vi "Main_2.vi"() -> ()   [LabVIEW 2016]
uses:
  <vilib>/Platform/TimedLoop/XDataNode/timing_clust.ctl
  <vilib>/Platform/TimedLoop/XDataNode/nitl_modes.ctl
  <vilib>/Platform/TimedLoop/XDataNode/wakeup.ctl
  <vilib>/Instr/_visa.llb/VISA Configure Serial Port (Instr).vi
  <vilib>/httpClient/POSTBuffer.vi
  <vilib>/platform/TimedLoop/XDataNode/XDataNode.xnode
  <vilib>/Platform/TimedLoop/XDataNode/XDNodeRunTimeDep.lvlib
  <vilib>/httpClient/LabVIEWHTTPClient.lvlib
panel:
  in  "?":enum32{"Battery", "Capacitor"}(tab)
  in  "?":enum32{"Rem Capacity", "Full Capacity"}(tab)
  out "BATTERY REM CAPACITY 4":dbl
  out "BATTERY REM CAPACITY 3":dbl
  out "BATTERY REM CAPACITY 2":dbl
  out "BATTERY REM CAPACITY 1":dbl
  out "BATTERY REM CAPACITY 5":dbl
  out "BATTERY FULL CAPACITY 4":dbl
  out "BATTERY FULL CAPACITY 3":dbl
  out "BATTERY FULL CAPACITY 2":dbl
  out "BATTERY FULL CAPACITY 1":dbl
  out "BATTERY FULL CAPACITY 5":dbl
  in  "?":T1(tab)
  out "BATTERY VOLTAGE 3":dbl
  out "BATTERY VOLTAGE 2":dbl
  out "BATTERY VOLTAGE 1":dbl
  out "BATTERY VOLTAGE 4":dbl
  out "Slide 4":u8(slide) scale=0.0..100.0
  out "Slide":u8(slide) scale=0.0..100.0
  out "Slide 2":u8(slide) scale=0.0..100.0
  out "Slide 3":u8(slide) scale=0.0..100.0
  out "BATTERY VOLTAGE 5":dbl
  out "Slide 8":u8(slide) scale=0.0..100.0
  out "Slide 7":u8(slide) scale=0.0..100.0
  out "Slide 6":u8(slide) scale=0.0..100.0
  out "Slide 5":u8(slide) scale=0.0..100.0
  out "BATTERY CURRENT 1":dbl
  out "BATTERY CURRENT 2":dbl
  out "BATTERY CURRENT 3":dbl
  out "BATTERY CURRENT 4":dbl
  out "BATTERY CURRENT 5":dbl
  in  "LO2-REL 2":bool
  in  "LO2-REL 1":bool
  in  "LO1-REL 2":bool
  in  "LO1-REL 1":bool
  in  "SUPERCAP-GATE 6":bool
  in  "BATT-GATE 4":bool
  in  "BATT-GATE 3":bool
  in  "BATT-GATE 5":bool
  in  "BATT-GATE 1":bool
  in  "BATT-GATE 2":bool
  out "Power Switch Led":bool
  out "Power Button State":dbl
  in  "Batter data send url":string
  in  "control battery url":string
  in  "VISA resource name":refnum<visa-resource-name>
  in  "Continuous Measurement":bool
  in  "?":enum32{"Temperature", "Power"}(tab)
  out "BATTERY TEMP: 4":dbl
  out "BATTERY TEMP: 3":dbl
  out "BATTERY TEMP: 2":dbl
  out "BATTERY TEMP: 1":dbl
  out "BATTERY TEMP: 5":dbl
  out "BATTERY POWER 5":dbl
  out "BATTERY POWER 4":dbl
  out "BATTERY  POWER 3":dbl
  out "BATTERY POWER 2":dbl
  out "BATTERY POWER 1":dbl
  in  "?":T2(tab)
  out "BATTERY RATED ENERGY 1":dbl
  out "BATTERY RATED ENERGY 2":dbl
  out "BATTERY RATED ENERGY 3":dbl
  out "BATTERY RATED ENERGY 4":dbl
  out "BATTERY RATED ENERGY 5":dbl
  out "BATTERY MAX ENERGY 4":dbl
  out "BATTERY MAX ENERGY 3":dbl
  out "BATTERY MAX ENERGY 2":dbl
  out "BATTERY MAX ENERGY 1":dbl
  out "BATTERY MAX ENERGY 5":dbl
  out "BATTERY AVAIL ENERGY 4":dbl
  out "BATTERY AVAIL ENERGY 3":dbl
  out "BATTERY AVAIL ENERGY 2":dbl
  out "BATTERY AVAIL ENERGY 1":dbl
  out "BATTERY AVAIL ENERGY 5":dbl
  in  "?":enum32{"Voltage", "Temperature", "TAP Voltage"}(tab)
  out "Vertical Progress Bar 6":u8(slide) scale=0.0..100.0
  out "Vertical Progress Bar 5":u8(slide) scale=0.0..100.0
  out "Vertical Progress Bar 4":u8(slide) scale=0.0..100.0
  out "Vertical Progress Bar 3":u8(slide) scale=0.0..100.0
  out "Vertical Progress Bar 2":u8(slide) scale=0.0..100.0
  out "Vertical Progress Bar":u8(slide) scale=0.0..100.0
  out "?":u8(slide) scale=0.0..100.0
  out "VOLT-CAP-6":dbl
  out "VOLT-CAP-5":dbl
  out "VOLT-CAP-4":dbl
  out "VOLT-CAP-3":dbl
  out "VOLT-CAP-2":dbl
  out "VOLT-CAP-1":dbl
  out "Temp_1":dbl(slide) scale=0.0..100.0
  out "Temp_2":dbl(slide) scale=0.0..100.0
  out "Temp_3":dbl(slide) scale=0.0..100.0
  out "Temp_4":dbl(slide) scale=0.0..100.0
  out "Temp_5":dbl(slide) scale=0.0..100.0
  out "Temp_6":dbl(slide) scale=0.0..100.0
  out "MOD 6":bool
  out "MOD 5":bool
  out "TAP 7":dbl(slide) scale=0.0..100.0
  out "TAP 8":dbl(slide) scale=0.0..100.0
  out "TAP 9":dbl(slide) scale=0.0..100.0
  out "TAP 10":dbl(slide) scale=0.0..100.0
  out "TAP 11":dbl(slide) scale=0.0..100.0
  out "TAP 12":dbl(slide) scale=0.0..100.0
  out "TAP 13":dbl(slide) scale=0.0..100.0
  out "TAP 14":dbl(slide) scale=0.0..100.0
  out "TAP 15":dbl(slide) scale=0.0..100.0
  out "TAP 16":dbl(slide) scale=0.0..100.0
  out "TAP 17":dbl(slide) scale=0.0..100.0
  out "TAP 18":dbl(slide) scale=0.0..100.0
  out "MOD 4":bool
  out "TAP 19":dbl(slide) scale=0.0..100.0
  out "TAP 20":dbl(slide) scale=0.0..100.0
  out "TAP 4_":dbl(slide) scale=0.0..100.0
  out "TAP 4_3":dbl(slide) scale=0.0..100.0
  out "TAP 4_2":dbl(slide) scale=0.0..100.0
  out "TAP 4_1":dbl(slide) scale=0.0..100.0
  out "MOD 3":bool
  out "MOD 2":bool
  out "MOD 1":bool
  out "TAP 3_3":dbl(slide) scale=0.0..12.0
  out "TAP 3_1":dbl(slide) scale=0.0..5.0
  out "TAP 3_2":dbl(slide) scale=0.0..8.0
  out "TAP 3_6":dbl(slide) scale=0.0..25.0
  out "TAP 3_4":dbl(slide) scale=0.0..16.0
  out "TAP 3_5":dbl(slide) scale=0.0..20.0
  out "TAP 2_6":dbl(slide) scale=0.0..25.0
  out "TAP 2_5":dbl(slide) scale=0.0..20.0
  out "TAP 2_4":dbl(slide) scale=0.0..16.0
  out "TAP 2_3":dbl(slide) scale=0.0..12.0
  out "TAP 2_2":dbl(slide) scale=0.0..8.0
  out "TAP 2_1":dbl(slide) scale=0.0..5.0
  out "TAP 1_5":dbl(slide) scale=0.0..20.0
  out "TAP 1_4":dbl(slide) scale=0.0..16.0
  out "TAP 1_6":dbl(slide) scale=0.0..25.0
  out "TAP 1_3":dbl(slide) scale=0.0..12.0
  out "TAP 1_2":dbl(slide) scale=0.0..8.0
  out "TAP 1_1":dbl(slide) scale=0.0..5.0
  in  "?":bool
  in  "Stop RT":bool
  out "TAP Voltages":cluster{dbl[], dbl[]}[](graph)
  out "Counter Register":dbl
  out "Total Received":u32
  out "Module's Voltages":cluster{dbl[], dbl[]}[](graph)
  in  "Transmit Frame":T3={"timestamp high"=0, "timestamp low"=0, "identifier"=18, "type"=enum."Data Frame", "info A"=0, "info B"=0, "data length"=8, "data"=[0, 0, 0, 0, 0, 0, 0, 0]} {"identifier" format="%x"; "data" format="%.0x"}
  # "https://aertcsmartgrid.onrender.com/receive-data"
  # "https://aertcsmartgrid.onrender.com/get-btcontrol"
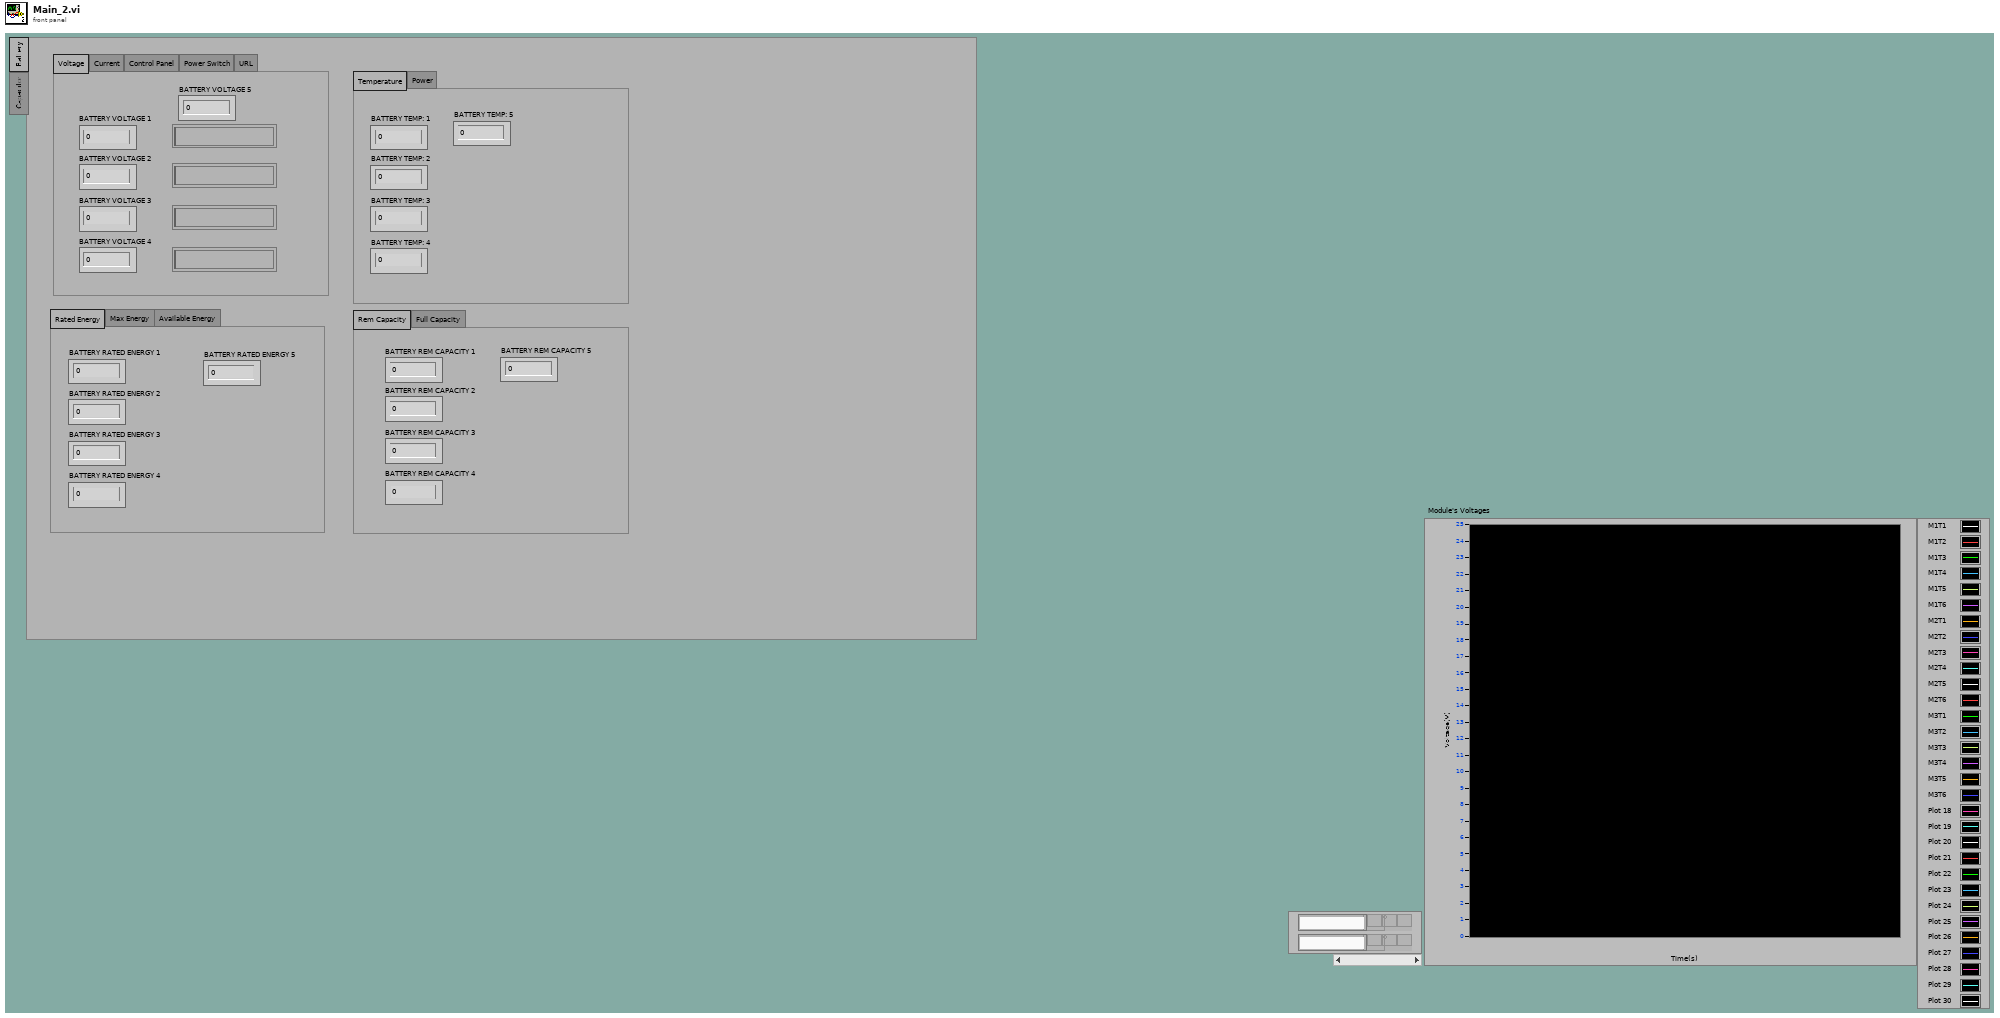
[diagram p1: front panel]
types:
  T1 = enum32{"Voltage", "Current", "Control Panel", "Power Switch", "URL"}
  T2 = enum32{"Rated Energy", "Max Energy", "Available Energy"}
  T3 = cluster{"timestamp high":u32, "timestamp low":u32, "identifier":u32, "type":enum8{"Data Frame", "Remote Frame", "(reserved)", "(reserved) ", "(reserved)  ", "(reserved)   ", "Bus Error", "Transceiver Fault"}, "info A":u8, "info B":u8, "data length":u8, "data":u8[]}
  T4 = typedef "XDNodeRunTimeDep.lvlib/timing_clust.ctl" = cluster{"Expected End [f-1]":u64, "Actual End [f-1]":u64, "Finished Late? [f-1]":bool, "Expected End [i-1]":u64, "Actual End [i-1]":u64, "Finished Late? [i-1]":bool, "Expected Start [i]":u64, "Actual Start [i]":u64, "Expected Start [f]":u64, "Actual Start [f]":u64, "Source Name":string, "Structure Name":string, "Period":i64, "Deadline":i64, "Offset":i64, "Start":i64, "Priority":i32, "Timeout":i32, "Mode":T5, "Wakeup Reason":T6, "Error":errorcluster, "Source Type":string, "Secondary Source Type":string, "Global End Time":u64, "Global Start Time":u64, "Frame Duration":u64, "Iteration Duration":u64, "Assigned CPU":i32, "I/O Scan Engine Mode":u32}
  T5 = typedef "XDNodeRunTimeDep.lvlib/nitl_modes.ctl" = enum32{"No Change", "Process missed periods, maintain original phase", "Discard missed periods, maintain original phase", "Process missed periods, ignore original phase", "Discard missed periods, ignore original phase"}
  T6 = typedef "XDNodeRunTimeDep.lvlib/wakeup.ctl" = enum32{"Normal", "Aborted", "Asynchronous wakeup", "Timing source error", "Timed loop error", "Timeout"}
  T7 = typedef "LabVIEWHTTPClient.lvlib/ClientHandle.ctl" = refnum<k1>
  T8 = cluster{"unsigned byte array[0]":u8, "unsigned byte array[1]":u8, "unsigned byte array[2]":u8, "unsigned byte array[3]":u8, "unsigned byte array[4]":u8, "unsigned byte array[5]":u8, "unsigned byte array[6]":u8, "unsigned byte array[7]":u8, "unsigned byte array[8]":u8}
  T9 = cluster{"data[0]":u8, "data[1]":u8, "data[2]":u8, "data[3]":u8, "data[4]":u8, "data[5]":u8, "data[6]":u8, "data[7]":u8, "data[8]":u8}
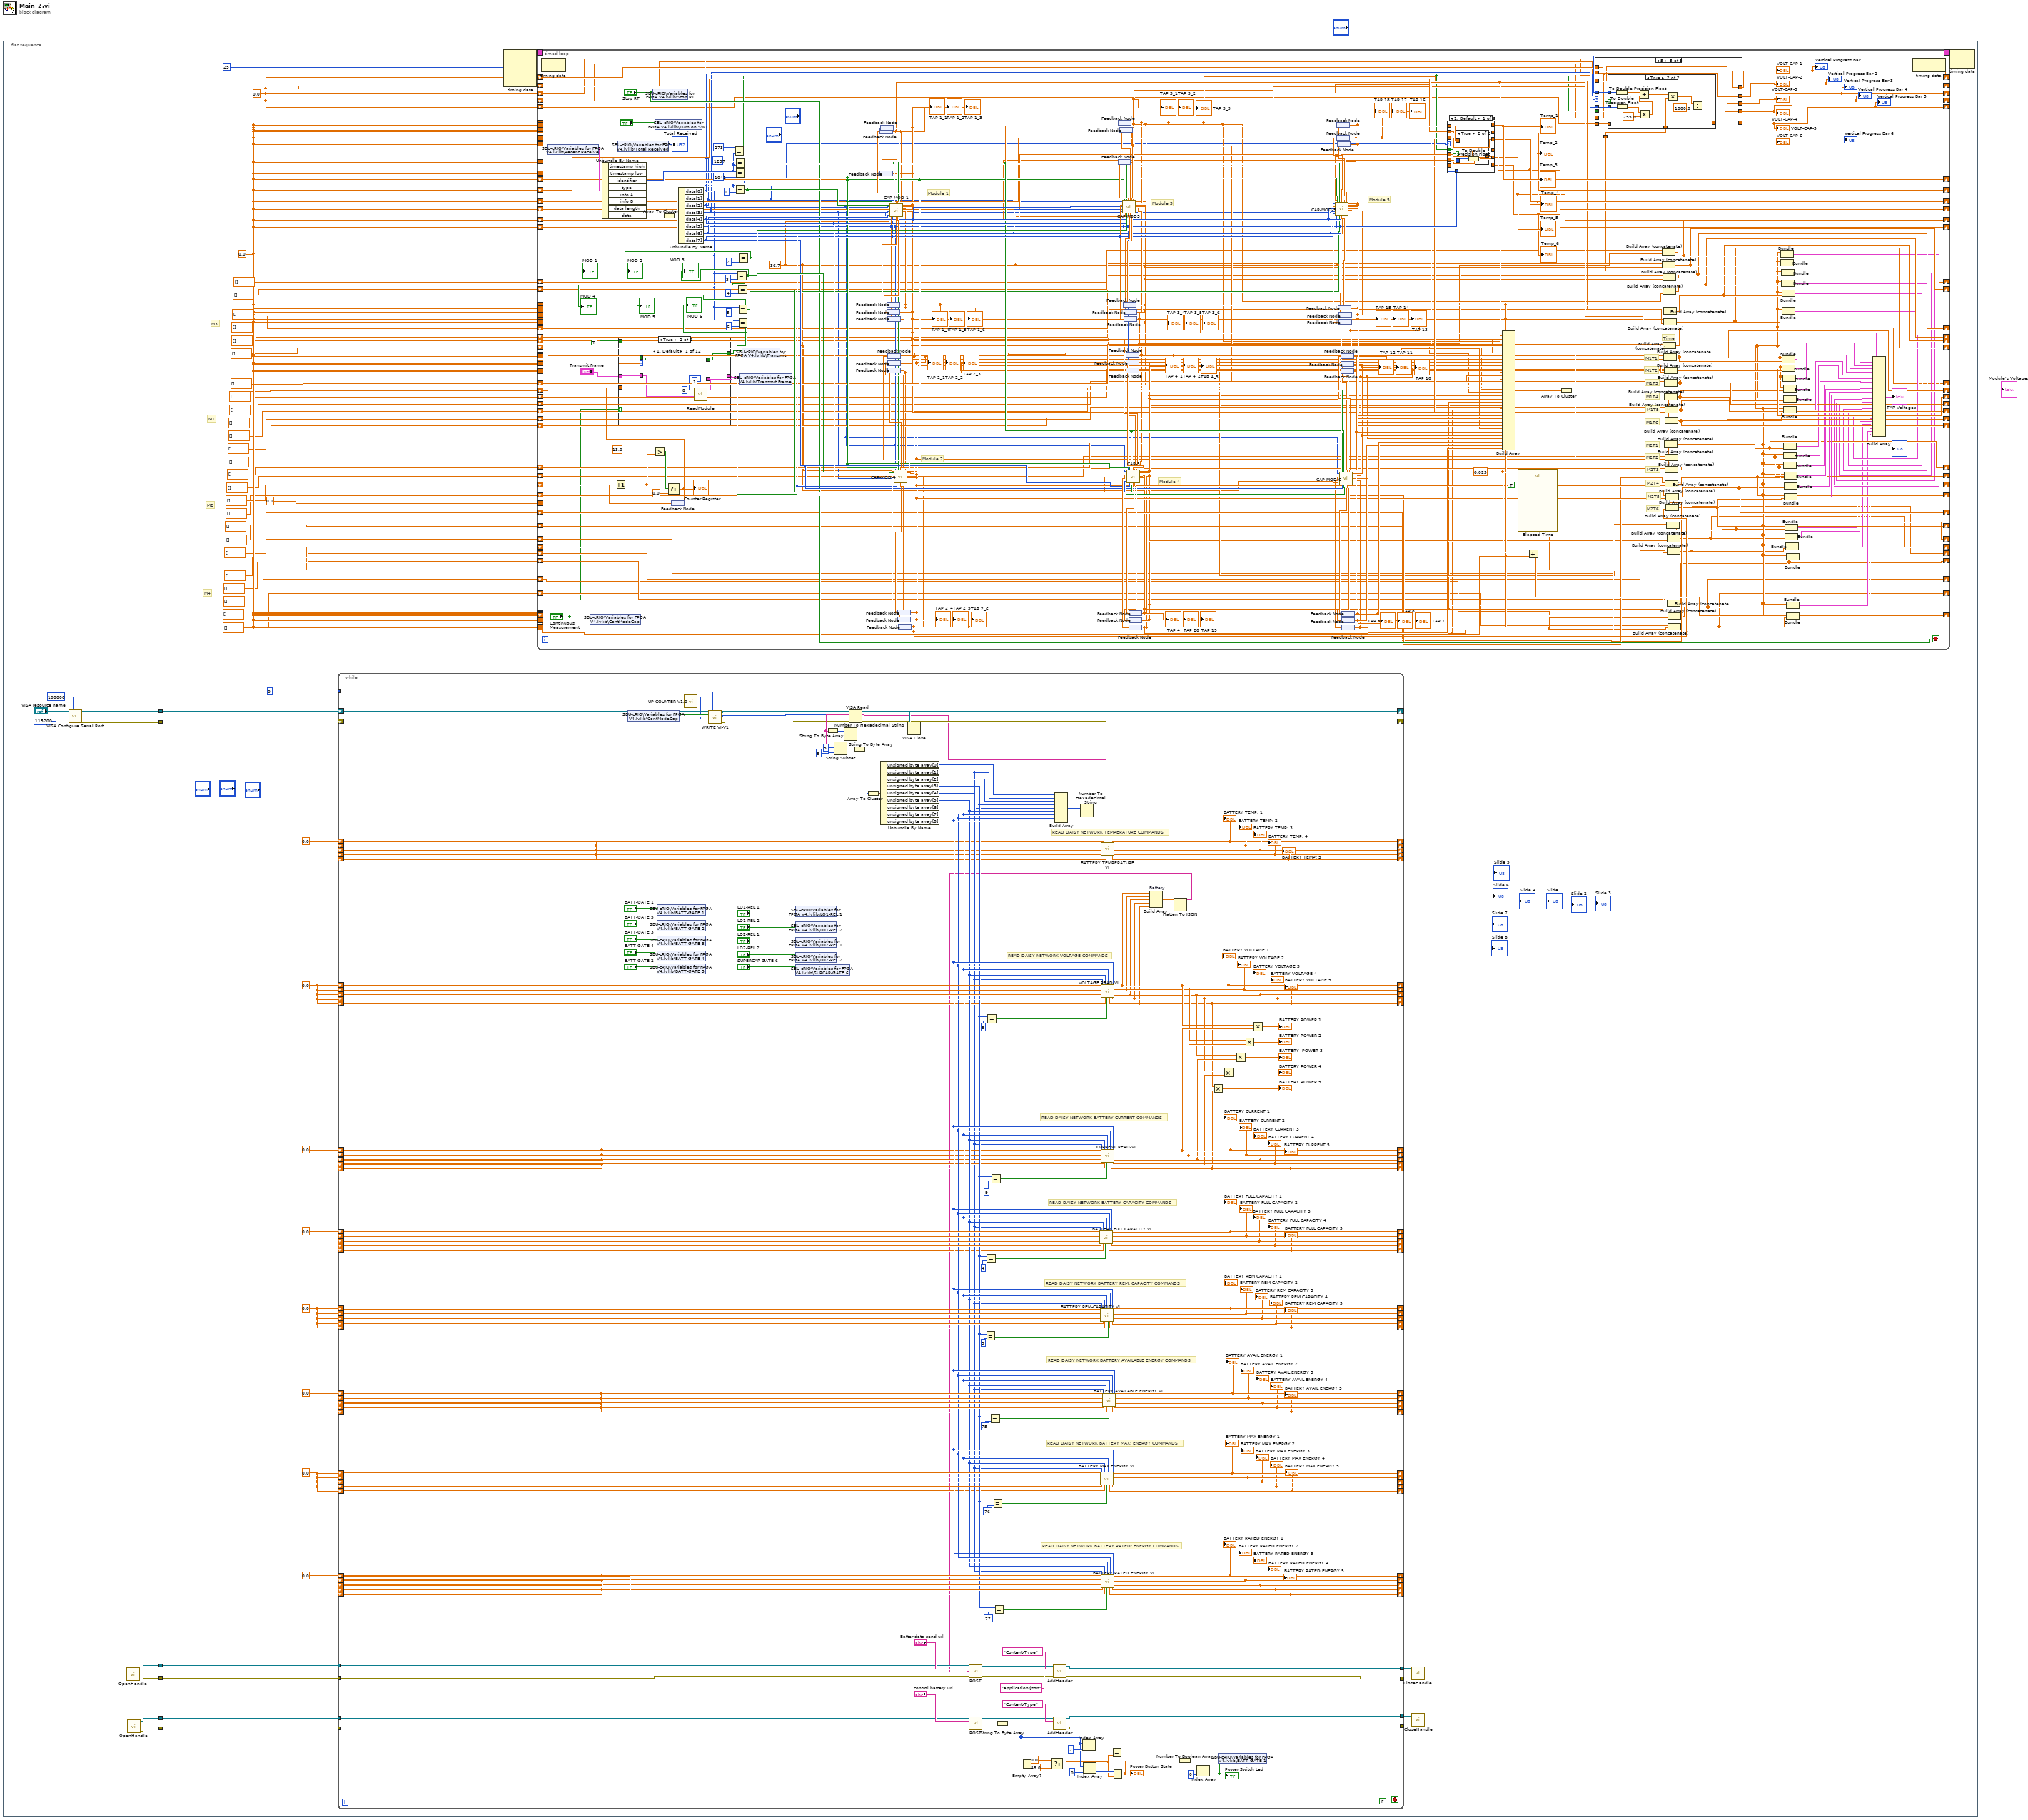
[diagram p0: block diagram]
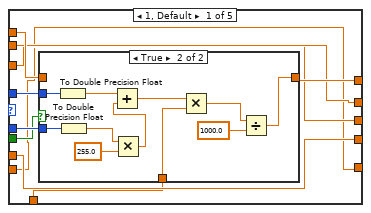
[diagram p2: hidden frame]
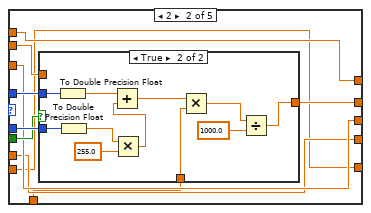
[diagram p4: hidden frame]
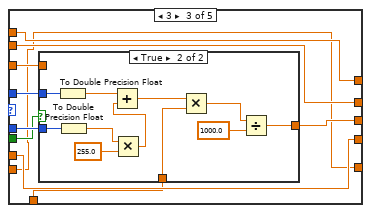
[diagram p6: hidden frame]
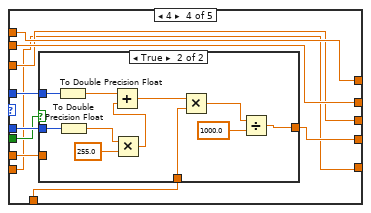
[diagram p8: hidden frame]
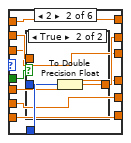
[diagram p12: hidden frame]
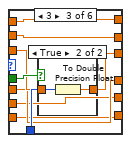
[diagram p14: hidden frame]
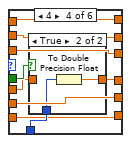
[diagram p16: hidden frame]
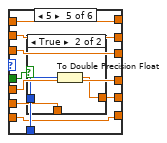
[diagram p18: hidden frame]
diagram:
  n1 = flat-sequence {
    tunnel: [w12] -> w6
    tunnel: [w11] -> w5
    tunnel: [w10] -> w4
    tunnel: [w9] -> w3
    tunnel: [w8] -> w2
    tunnel: [w7] -> w1
    tunnel: w6 -> [w34]
    tunnel: w5 -> [w33]
    tunnel: w4 -> [w19]
    tunnel: w3 -> [w18]
    tunnel: w2 -> [w17]
    tunnel: w1 -> [w16]
    frame #0 {
      n2 = call-poly "VISA Configure Serial Port"("VISA resource name"="VISA resource name", "timeout (10sec)"=u32 100000, "baud rate (9600)"=u32 115200) -> ("VISA resource name out"=w12:refnum<visa-resource-name>, "error out"=w11:errorcluster)  [unwired: 11 in]
      n3 = call <vilib>:"OpenHandle.vi"() -> ("client handle out"=w10:T7, "error out"=w9:errorcluster)  [unwired: 14 in]
      n4 = call <vilib>:"OpenHandle.vi"() -> ("client handle out"=w8:T7, "error out"=w7:errorcluster)  [unwired: 14 in]
    }
    frame #1 {
      w30 = 0.0
      w24 = 0.0
      w32 = 0.0
      w27 = 0.0
      w26 = 0.0
      w28 = 0.0
      w25 = 0.0
      w29 = 0.0
      w31 = 0.0
      w62 = 0.0
      # "M4"
      # "M3"
      # "M2"
      # "M1"
      n5 = while {
        shift-right: [w117] -> w37
        shift-left: w34 -> [w75]
        shift-right: [w116] -> w36
        shift-left: w33 -> [w69]
        tunnel: 0 -> [w73]
        shift-right: [w82] -> _
        shift-left: w31 -> [w173]
        shift-right: [w81] -> _
        shift-left: w31 -> [w174]
        shift-right: [w80] -> _
        shift-left: w31 -> [w175]
        shift-right: [w79] -> _
        shift-left: w31 -> [w176]
        shift-right: [w215] -> _
        shift-left: w29 -> [w216]
        shift-right: [w214] -> _
        shift-left: w29 -> [w172]
        shift-right: [w213] -> _
        shift-left: w29 -> [w211]
        shift-right: [w212] -> _
        shift-left: w29 -> [w210]
        shift-right: [w205] -> _
        shift-left: w25 -> [w209]
        shift-right: [w204] -> _
        shift-left: w25 -> [w208]
        shift-right: [w203] -> _
        shift-left: w25 -> [w207]
        shift-right: [w202] -> _
        shift-left: w25 -> [w206]
        shift-right: [w201] -> _
        shift-left: w28 -> [w197]
        shift-right: [w200] -> _
        shift-left: w28 -> [w196]
        shift-right: [w199] -> _
        shift-left: w28 -> [w195]
        shift-right: [w198] -> _
        shift-left: w28 -> [w194]
        shift-right: [w189] -> _
        shift-left: w26 -> [w193]
        shift-right: [w188] -> _
        shift-left: w26 -> [w192]
        shift-right: [w187] -> _
        shift-left: w26 -> [w191]
        shift-right: [w186] -> _
        shift-left: w26 -> [w190]
        shift-right: [w181] -> _
        shift-left: w27 -> [w185]
        shift-right: [w180] -> _
        shift-left: w27 -> [w184]
        shift-right: [w179] -> _
        shift-left: w27 -> [w183]
        shift-right: [w178] -> _
        shift-left: w27 -> [w182]
        shift-right: [w160] -> _
        shift-left: w30 -> [w163]
        shift-right: [w158] -> _
        shift-left: w30 -> [w162]
        shift-right: [w157] -> _
        shift-left: w30 -> [w161]
        shift-right: [w156] -> _
        shift-left: w30 -> [w164]
        shift-right: [w78] -> _
        shift-left: w31 -> [w152]
        shift-right: [w148] -> _
        shift-left: w30 -> [w150]
        shift-right: [w146] -> _
        shift-left: w29 -> [w147]
        shift-right: [w144] -> _
        shift-left: w25 -> [w145]
        shift-right: [w142] -> _
        shift-left: w28 -> [w143]
        shift-right: [w140] -> _
        shift-left: w26 -> [w141]
        shift-right: [w138] -> _
        shift-left: w27 -> [w139]
        shift-right: [w132] -> _
        shift-left: w24 -> [w137]
        shift-right: [w131] -> _
        shift-left: w24 -> [w136]
        shift-right: [w130] -> _
        shift-left: w24 -> [w135]
        shift-right: [w129] -> _
        shift-left: w24 -> [w134]
        shift-right: [w114] -> _
        shift-left: w24 -> [w133]
        tunnel: [w91] -> w23
        tunnel: [w90] -> w22
        tunnel: [w89] -> w21
        tunnel: [w88] -> w20
        tunnel: w19 -> [w87]
        tunnel: w18 -> [w86]
        tunnel: w17 -> [w85]
        tunnel: w16 -> [w84]
        stop <- FALSE stop-if-true
        # "READ DAISY NETWORK TEMPERATURE COMMANDS"
        # "READ DAISY NETWORK BATTERY CURRENT COMMANDS"
        # "READ DAISY NETWORK BATTERY RATED: ENERGY COMMANDS"
        # "READ DAISY NETWORK BATTERY MAX: ENERGY COMMANDS"
        # "READ DAISY NETWORK BATTERY AVAILABLE ENERGY COMMANDS"
        # "READ DAISY NETWORK BATTERY REM: CAPACITY COMMANDS"
        # "READ DAISY NETWORK BATTERY CAPACITY COMMANDS"
        # "READ DAISY NETWORK VOLTAGE COMMANDS"
        n6 = shared-variable "SBU-cRIO\\Variables for FPGA V4.lvlib\\ContModeCap"() -> (w72:bool)  [unwired: 1 in, 1 out]
        n7 = shared-variable "SBU-cRIO\\Variables for FPGA V4.lvlib\\BATT-GATE 1"("BATT-GATE 1") -> ()  [unwired: 1 in, 1 out]
        n8 = shared-variable "SBU-cRIO\\Variables for FPGA V4.lvlib\\BATT-GATE 2"("BATT-GATE 5") -> ()  [unwired: 1 in, 1 out]
        n9 = shared-variable "SBU-cRIO\\Variables for FPGA V4.lvlib\\BATT-GATE 3"("BATT-GATE 3") -> ()  [unwired: 1 in, 1 out]
        n10 = shared-variable "SBU-cRIO\\Variables for FPGA V4.lvlib\\BATT-GATE 4"("BATT-GATE 4") -> ()  [unwired: 1 in, 1 out]
        n11 = shared-variable "SBU-cRIO\\Variables for FPGA V4.lvlib\\BATT-GATE 5"("BATT-GATE 2") -> ()  [unwired: 1 in, 1 out]
        n12 = call "UP-COUNTER-V1.0.vi"() -> ("COUNT"=w68:u32)  [unwired: 11 in]
        n13 = call "WRITE VI-V1.vi"("Numeric"=w73, "error in (no error)"=w69, "COUNT"=w68, "BATTERY MEASUREMENTS"=w72, "VISA Refnum in"=w75) -> ("error out"=w70:errorcluster, "Bytes at Port"=w71:u32, "VISA Refnum out"=w74:refnum<visa-resource-name>)  [unwired: 4 in]
        n14 = shared-variable "SBU-cRIO\\Variables for FPGA V4.lvlib\\LO1-REL 1"("LO1-REL 1") -> ()  [unwired: 1 in, 1 out]
        n15 = shared-variable "SBU-cRIO\\Variables for FPGA V4.lvlib\\LO1-REL 2"("LO1-REL 2") -> ()  [unwired: 1 in, 1 out]
        n16 = shared-variable "SBU-cRIO\\Variables for FPGA V4.lvlib\\LO2-REL 1"("LO2-REL 1") -> ()  [unwired: 1 in, 1 out]
        n17 = shared-variable "SBU-cRIO\\Variables for FPGA V4.lvlib\\LO2-REL 2"("LO2-REL 2") -> ()  [unwired: 1 in, 1 out]
        n18 = shared-variable "SBU-cRIO\\Variables for FPGA V4.lvlib\\SUPCAP-GATE 6"("SUPERCAP-GATE 6") -> ()  [unwired: 1 in, 1 out]
        n19 = VISA Read(VISA resource name=w74, byte count=w71, error in (no error)=w70) -> (VISA resource name out=w117:refnum<visa-resource-name>, read buffer=w115:string, error out=w116:errorcluster)  [unwired: 1 out]
        n20 = String To Byte Array(string=w115) -> (unsigned byte array=w217:u8[])
        n21 = String Subset(string=w115, offset (0)=5, length (rest)=8 ("length (rest)")) -> (substring=w234:string)
        n22 = Number To Hexadecimal String(2:w217) -> ()  [unwired: 1 in, 1 out]
        n23 = String To Byte Array(string=w234) -> (unsigned byte array=w233:u8[])
        n24 = Array To Cluster(array=w233) -> (cluster=w229:T8)
        n25 = Unbundle By Name(w229) -> ("unsigned byte array[0]"=w232:u8, "unsigned byte array[1]"=w151:u8, "unsigned byte array[2]"=w231:u8, "unsigned byte array[3]"=w165:u8, "unsigned byte array[4]"=w118:u8, "unsigned byte array[5]"=w166:u8, "unsigned byte array[6]"=w167:u8, "unsigned byte array[7]"=w168:u8, "unsigned byte array[8]"=w169:u8)
        n26 = call-poly <vilib>:"POST.vi"("client handle"=w85, "url"="control battery url", "error in (no error)"=w84) -> ("client handle out"=w106:T7, "body"=w102:string, "error out"=w105:errorcluster)  [unwired: 9 in, 1 out]
        n27 = Equal?(x=w165, y=u32 3) -> (x = y?=w224:bool)
        n28 = Equal?(x=w165, y=u32 4) -> (x = y?=w226:bool)
        n29 = Equal?(x=w165, y=u32 8) -> (x = y?=w177:bool)
        n30 = Equal?(x=w165, y=u32 75) -> (x = y?=w222:bool)
        n31 = Equal?(x=w165, y=u32 9) -> (x = y?=w170:bool)
        n32 = Equal?(x=w165, y=u32 76) -> (x = y?=w220:bool)
        n33 = Equal?(x=w165, y=u32 77) -> (x = y?=w218:bool)
        n34 = String To Byte Array(string=w102) -> (unsigned byte array=w98:u8[])
        n35 = Empty Array?(array=w98) -> (empty?=w99:bool)
        n36 = Select(t=0.0 ("x"), s=w99, f=48.0 ("x")) -> (s? t:f=w95:dbl)
        n37 = call <vilib>:"AddHeader.vi"("client handle"=w106, "header"="Content-Type", "error in (no error)"=w105) -> ("client handle out"=w89:T7, "error out"=w88:errorcluster)  [unwired: 11 in]
        n38 = Build Array(w232, w151, w231, w165, w118, w166, w167, w168, w169) -> (w230:u8[])
        n39 = Number To Hexadecimal String(2:w230) -> ()  [unwired: 1 in, 1 out]
        n40 = Index Array(array=w98, index=2) -> (element=w101:u8)
        n41 = Index Array(array=w98, index=0) -> (element=w100:u8)
        n42 = call "BATTERY FULL CAPACITY VI.vi"("unsigned byte array[7]"=w168, "unsigned byte array[6]"=w167, "unsigned byte array[5]"=w166, "unsigned byte array[1]"=w151, "unsigned byte array[8]"=w169, "Numeric 4"=w216, "Numeric 3"=w172, "Numeric 5"=w147, "Numeric 2"=w211, "Numeric"=w210, "Boolean"=w226) -> ("Numeric 9"=w215:dbl, "Numeric 8"=w214:dbl, "Numeric 7"=w213:dbl, "Numeric 6"=w212:dbl, "Numeric 10"=w146:dbl)
        "BATTERY FULL CAPACITY 1" <- w215
        "BATTERY FULL CAPACITY 2" <- w214
        "BATTERY FULL CAPACITY 3" <- w213
        "BATTERY FULL CAPACITY 4" <- w212
        "BATTERY FULL CAPACITY 5" <- w146
        n43 = call "BATTERY REM-CAPACITY VI.vi"("unsigned byte array[7]"=w168, "unsigned byte array[6]"=w167, "unsigned byte array[5]"=w166, "unsigned byte array[1]"=w151, "unsigned byte array[8]"=w169, "Numeric 9"=w209, "Numeric 8"=w208, "Numeric 10"=w145, "Boolean"=w224, "Numeric 7"=w207, "Numeric 6"=w206) -> ("Numeric 4"=w205:dbl, "Numeric 3"=w204:dbl, "Numeric 2"=w203:dbl, "Numeric"=w202:dbl, "Numeric 5"=w144:dbl)
        "BATTERY REM CAPACITY 1" <- w205
        "BATTERY REM CAPACITY 2" <- w204
        "BATTERY REM CAPACITY 3" <- w203
        "BATTERY REM CAPACITY 4" <- w202
        "BATTERY REM CAPACITY 5" <- w144
        n44 = call "BATTERY MAX ENERGY VI.vi"("unsigned byte array[7]"=w168, "unsigned byte array[6]"=w167, "unsigned byte array[5]"=w166, "unsigned byte array[1]"=w151, "unsigned byte array[8]"=w169, "Numeric 9"=w193, "Numeric 8"=w192, "Numeric 10"=w141, "Boolean"=w220, "Numeric 7"=w191, "Numeric 6"=w190) -> ("Numeric 4"=w189:dbl, "Numeric 3"=w188:dbl, "Numeric 2"=w187:dbl, "Numeric"=w186:dbl, "Numeric 5"=w140:dbl)
        "BATTERY MAX ENERGY 1" <- w189
        "BATTERY MAX ENERGY 2" <- w188
        "BATTERY MAX ENERGY 3" <- w187
        "BATTERY MAX ENERGY 4" <- w186
        "BATTERY MAX ENERGY 5" <- w140
        n45 = call "BATTERY TEMPERATURE VI.vi"("Numeric Control in"=w137, "Numeric Control 6"=w136, "read buffer"=w115, "Numeric Control 7"=w135, "Numeric Control 8"=w134, "Numeric Control 9"=w133) -> ("Numeric Control out"=w132:dbl, "Numeric Control 4"=w130:dbl, "Numeric Control 5"=w129:dbl, "Numeric Control 10"=w114:dbl, "Numeric Control 3"=w131:dbl)  [unwired: 1 in]
        "BATTERY TEMP: 1" <- w114
        "BATTERY TEMP: 2" <- w129
        "BATTERY TEMP: 3" <- w130
        "BATTERY TEMP: 4" <- w131
        "BATTERY TEMP: 5" <- w132
        n46 = call "VOLTAGE READ-VI.vi"("unsigned byte array[7]"=w168, "unsigned byte array[6]"=w167, "unsigned byte array[5]"=w166, "unsigned byte array[1]"=w151, "unsigned byte array[8]"=w169, "Numeric 8"=w173, "Numeric 7"=w174, "Numeric 9"=w152, "Numeric 6"=w175, "Numeric 5"=w176, "Boolean"=w177) -> ("Numeric 4"=w82:dbl, "Numeric 3"=w81:dbl, "Numeric 2"=w80:dbl, "Numeric"=w79:dbl, "Numeric 10"=w78:dbl)
        "BATTERY VOLTAGE 4" <- w79
        "BATTERY VOLTAGE 1" <- w82
        "BATTERY VOLTAGE 2" <- w81
        "BATTERY VOLTAGE 3" <- w80
        "BATTERY VOLTAGE 5" <- w78
        n47 = call "CURRENT READ-VI.vi"("unsigned byte array[7]"=w168, "unsigned byte array[6]"=w167, "unsigned byte array[5]"=w166, "unsigned byte array[1]"=w151, "unsigned byte array[8]"=w169, "Numeric 4"=w163, "Numeric 3"=w162, "Numeric 5"=w150, "Boolean"=w170, "Numeric 2"=w161, "Numeric"=w164) -> ("Numeric 9"=w160:dbl, "Numeric 8"=w158:dbl, "Numeric 7"=w157:dbl, "Numeric 6"=w156:dbl, "Numeric 10"=w148:dbl)
        "BATTERY CURRENT 1" <- w160
        "BATTERY CURRENT 2" <- w158
        "BATTERY CURRENT 3" <- w157
        "BATTERY CURRENT 4" <- w156
        "BATTERY CURRENT 5" <- w148
        n48 = call "BATTERY RATED ENERGY VI.vi"("unsigned byte array[7]"=w168, "unsigned byte array[6]"=w167, "unsigned byte array[5]"=w166, "unsigned byte array[1]"=w151, "unsigned byte array[8]"=w169, "Boolean"=w218, "Numeric 9"=w185, "Numeric 10"=w139, "Numeric 8"=w184, "Numeric 7"=w183, "Numeric 6"=w182) -> ("Numeric 4"=w181:dbl, "Numeric 3"=w180:dbl, "Numeric 2"=w179:dbl, "Numeric"=w178:dbl, "Numeric 5"=w138:dbl)
        "BATTERY RATED ENERGY 1" <- w181
        "BATTERY RATED ENERGY 2" <- w180
        "BATTERY RATED ENERGY 3" <- w179
        "BATTERY RATED ENERGY 4" <- w178
        "BATTERY RATED ENERGY 5" <- w138
        n49 = call "BATTERY AVAILABLE ENERGY VI.vi"("unsigned byte array[7]"=w168, "unsigned byte array[6]"=w167, "unsigned byte array[5]"=w166, "unsigned byte array[1]"=w151, "unsigned byte array[8]"=w169, "Numeric 4"=w197, "Numeric 3"=w196, "Numeric 5"=w143, "Boolean"=w222, "Numeric 2"=w195, "Numeric"=w194) -> ("Numeric 9"=w201:dbl, "Numeric 8"=w200:dbl, "Numeric 7"=w199:dbl, "Numeric 6"=w198:dbl, "Numeric 10"=w142:dbl)
        "BATTERY AVAIL ENERGY 1" <- w201
        "BATTERY AVAIL ENERGY 2" <- w200
        "BATTERY AVAIL ENERGY 3" <- w199
        "BATTERY AVAIL ENERGY 4" <- w198
        "BATTERY AVAIL ENERGY 5" <- w142
        n50 = Subtract(x=w101, y=w95) -> ()  [unwired: 1 out]
        n51 = Subtract(x=w100, y=w95) -> (x-y=w94:dbl)
        "Power Button State" <- w94
        n52 = Build Array "Battery"(w82, w81, w80, w79, w78) -> (w83:dbl[])
        n53 = Flatten To JSON(anything=w83) -> (JSON string=w77:string)  [unwired: 2 in, 1 out]
        n54 = call-poly <vilib>:"POST.vi"("client handle"=w87, "url"="Batter data send url", "buffer"=w77, "error in (no error)"=w86) -> ("client handle out"=w110:T7, "error out"=w109:errorcluster)  [unwired: 8 in, 2 out]
        n55 = call <vilib>:"AddHeader.vi"("client handle"=w110, "header"="Content-Type", "value"="application/json", "error in (no error)"=w109) -> ("client handle out"=w91:T7, "error out"=w90:errorcluster)  [unwired: 10 in]
        n56 = Number To Boolean Array(number=w94) -> (Boolean array=w93:bool[])
        n57 = Index Array(array=w93, index=0) -> (element=w76:bool)
        "Power Switch Led" <- w76
        n58 = Multiply(x=w78, y=w148) -> (x*y=→"BATTERY POWER 5":dbl)
        n59 = shared-variable "SBU-cRIO\\Variables for FPGA V4.lvlib\\BATT-GATE 1"(w76) -> ()  [unwired: 1 in, 1 out]
        n60 = Multiply(x=w79, y=w156) -> (x*y=→"BATTERY POWER 4":dbl)
        n61 = Multiply(x=w80, y=w157) -> (x*y=→"BATTERY  POWER 3":dbl)
        n62 = Multiply(x=w81, y=w158) -> (x*y=→"BATTERY POWER 2":dbl)
        n63 = Multiply(x=w82, y=w160) -> (x*y=→"BATTERY POWER 1":dbl)
      }
      n64 = node-c288(i64 25 ("Period")) -> (w67:T4)  [unwired: 3 in]
      n65 = timed-loop "Timed loop" {
        timing: w67 -> [_]
        timing-out: [_] -> w66
        border: w62 -> [_]
        border: w62 -> [_]
        border: w62 -> [_]
        border: w62 -> [_]
        border: w62 -> [_]
        border: w62 -> [_]
        border: 0.0 -> [_]
        border: w62 -> [_]
        border: w62 -> [_]
        border: w62 -> [_]
        border: w62 -> [_]
        border: w62 -> [_]
        border: w62 -> [_]
        border: w62 -> [_]
        border: w62 -> [_]
        border: w62 -> [_]
        border: w62 -> [_]
        border: w62 -> [_]
        border: w62 -> [_]
        border: w62 -> [_]
        border: w62 -> [_]
        border: w62 -> [_]
        border: w62 -> [_]
        border: w62 -> [_]
        border: w62 -> [_]
        border: w62 -> [_]
        border: w62 -> [_]
        border: w62 -> [_]
        border: w62 -> [_]
        border: w62 -> [_]
        border: w62 -> [_]
        border: w62 -> [_]
        border: w62 -> [_]
        border: w62 -> [_]
        border: w62 -> [_]
        border: w62 -> [_]
        border: w62 -> [_]
        shift-right: [w385] -> _
        shift-left: w62 -> [w384]
        shift-right: [w380] -> _
        shift-left: w62 -> [w379]
        shift-right: [w377] -> _
        shift-left: w62 -> [w378]
        shift-right: [w375] -> _
        shift-left: w62 -> [w376]
        shift-right: [w374] -> _
        shift-left: w62 -> [w373]
        shift-right: [w372] -> _
        shift-left: w62 -> [w371]
        shift-right: [w353] -> _
        shift-left: w62 -> [w352]
        shift-right: [w279] -> _
        shift-left: dbl[] [] -> [w356]
        shift-right: [w333] -> _
        shift-left: dbl[] [] -> [w350]
        shift-right: [w332] -> _
        shift-left: dbl[] [] -> [w344]
        shift-right: [w331] -> _
        shift-left: dbl[] [] -> [w343]
        shift-right: [w330] -> _
        shift-left: dbl[] [] -> [w342]
        shift-right: [w329] -> _
        shift-left: dbl[] [] -> [w341]
        shift-right: [w328] -> _
        shift-left: dbl[] [] -> [w340]
        shift-right: [w306] -> _
        shift-left: dbl[] [] -> [w312]
        shift-right: [w305] -> _
        shift-left: dbl[] [] -> [w311]
        shift-right: [w309] -> _
        shift-left: dbl[] [] -> [w315]
        shift-right: [w308] -> _
        shift-left: dbl[] [] -> [w314]
        shift-right: [w307] -> _
        shift-left: dbl[] [] -> [w313]
        shift-right: [w304] -> _
        shift-left: dbl[] [] -> [w310]
        shift-right: [w291] -> _
        shift-left: dbl[] [] -> [w297]
        shift-right: [w290] -> _
        shift-left: dbl[] [] -> [w296]
        shift-right: [w289] -> _
        shift-left: dbl[] [] -> [w295]
        shift-right: [w288] -> _
        shift-left: dbl[] [] -> [w294]
        shift-right: [w287] -> _
        shift-left: dbl[] [] -> [w293]
        shift-right: [w286] -> _
        shift-left: dbl[] [] -> [w292]
        shift-right: [w260] -> _
        shift-left: dbl[] [] -> [w272]
        shift-right: [w259] -> _
        shift-left: dbl[] [] -> [w271]
        shift-right: [w258] -> _
        shift-left: dbl[] [] -> [w270]
        shift-right: [w261] -> _
        shift-left: dbl[] [] -> [w273]
        shift-right: [w257] -> _
        shift-left: dbl[] [] -> [w269]
        shift-right: [w256] -> _
        shift-left: dbl[] [] -> [w268]
        shift-right: [w243] -> _
        shift-left: w32 -> [w251]
        shift-right: [w242] -> _
        shift-left: w32 -> [w250]
        shift-right: [w241] -> _
        shift-left: w32 -> [w249]
        shift-right: [w240] -> _
        shift-left: w32 -> [w248]
        shift-right: [w239] -> _
        shift-left: w32 -> [w246]
        stop <- "Stop RT" stop-if-true
        w247 = 36.7 ("Count per volt")
        w354 = 0.025 ("Time Target (s)")
        # "Module 1"
        # "Module 2"
        # "Module 3"
        # "Module 4"
        # "Module 5"
        # "M2T6"
        # "M2T5"
        # "M2T4"
        # "M2T3"
        # "M2T2"
        # "M2T1"
        # "M1T6"
        # "M1T5"
        # "M1T4"
        # "M1T3"
        # "M1T2"
        # "M1T1"
        # "M1T1"
        # "Time"
        n66 = node-c288() -> ()  [unwired: 1 in, 1 out]
        n67 = shared-variable "SBU-cRIO\\Variables for FPGA V4.lvlib\\Recent Receive"() -> (w444:T3)  [unwired: 1 in, 1 out]
        n68 = shared-variable "SBU-cRIO\\Variables for FPGA V4.lvlib\\ContModeCap"("Continuous Measurement") -> ()  [unwired: 1 in, 1 out]
        n69 = Unbundle By Name(w444) -> ("identifier"=w387:u32, "data"=w443:u8[])  [unwired: 6 out]
        n70 = shared-variable "SBU-cRIO\\Variables for FPGA V4.lvlib\\Total Received"() -> (→"Total Received":u32)  [unwired: 1 in, 1 out]
        n71 = shared-variable "SBU-cRIO\\Variables for FPGA V4.lvlib\\Stop RT"("Stop RT") -> ()  [unwired: 1 in, 1 out]
        n72 = shared-variable "SBU-cRIO\\Variables for FPGA V4.lvlib\\Turn on SW1"("?") -> ()  [unwired: 1 in, 1 out]
        n73 = Array To Cluster(array=w443) -> (cluster=w446:T9)
        n74 = feedback #1() -> (w450:dbl)
        n75 = Increment(x=w450) -> (x+1=w449:dbl)
        n76 = Greater?(x=13.0, y=w449) -> (0:w451:bool)
        n77 = Select(t=w449, s=w451, f=0.0 ("t")) -> (s? t:f=w383:dbl)
        "Counter Register" <- w383
        n78 = case shown="True" "Continuous Measurement" {
          tunnel: "Transmit Frame" -> [w639 w644]
          tunnel: [w639 w643] -> w453
          tunnel: w383 -> [_ w642]
          tunnel: TRUE -> [w638 w641]
          tunnel: [w638 w640] -> w447
          frame False {
          }
          frame True {
            n79 = case shown="1, Default" w642 {
              tunnel: w644 -> [w647 w654 w659 w664 w669 w674 w679 w684 w689 w694 w699 w704]
              tunnel: [w646 w653 w658 w663 w668 w673 w678 w683 w688 w693 w698 w703] -> w643
              tunnel: w641 -> [w645 w650 w655 w660 w665 w670 w675 w680 w685 w690 w695 w700]
              tunnel: [w645 w650 w655 w660 w665 w670 w675 w680 w685 w690 w695 w700] -> w640
              frame 1, Default {
                n80 = call "ReadModule.vi"("Transmit Frame in"=w647, "Numeric"=8, "Numeric 2"=1) -> ("Transmit Frame out"=w646:T3)  [unwired: 8 in]
              }
              frame 2 {
                n81 = call "ReadModule.vi"("Transmit Frame in"=w654, "Numeric"=8, "Numeric 2"=2) -> ("Transmit Frame out"=w653:T3)  [unwired: 8 in]
              }
              frame 3 {
                n82 = call "ReadModule.vi"("Transmit Frame in"=w659, "Numeric"=8, "Numeric 2"=3) -> ("Transmit Frame out"=w658:T3)  [unwired: 8 in]
              }
              frame 4 {
                n83 = call "ReadModule.vi"("Transmit Frame in"=w664, "Numeric"=8, "Numeric 2"=4) -> ("Transmit Frame out"=w663:T3)  [unwired: 8 in]
              }
              frame 5 {
                n84 = call "ReadModule.vi"("Transmit Frame in"=w669, "Numeric"=8, "Numeric 2"=5) -> ("Transmit Frame out"=w668:T3)  [unwired: 8 in]
              }
              frame 6 {
                n85 = call "ReadModule.vi"("Transmit Frame in"=w674, "Numeric"=8, "Numeric 2"=6) -> ("Transmit Frame out"=w673:T3)  [unwired: 8 in]
              }
              frame 7 {
                n86 = call "ReadModule.vi"("Transmit Frame in"=w679, "Numeric"=1, "Numeric 2"=1) -> ("Transmit Frame out"=w678:T3)  [unwired: 8 in]
              }
              frame 8 {
                n87 = call "ReadModule.vi"("Transmit Frame in"=w684, "Numeric"=1, "Numeric 2"=2) -> ("Transmit Frame out"=w683:T3)  [unwired: 8 in]
              }
              frame 9 {
                n88 = call "ReadModule.vi"("Transmit Frame in"=w689, "Numeric"=1, "Numeric 2"=3) -> ("Transmit Frame out"=w688:T3)  [unwired: 8 in]
              }
              frame 10 {
                n89 = call "ReadModule.vi"("Transmit Frame in"=w694, "Numeric"=1, "Numeric 2"=4) -> ("Transmit Frame out"=w693:T3)  [unwired: 8 in]
              }
              frame 11 {
                n90 = call "ReadModule.vi"("Transmit Frame in"=w699, "Numeric"=1, "Numeric 2"=5) -> ("Transmit Frame out"=w698:T3)  [unwired: 8 in]
              }
              frame 12 {
                n91 = call "ReadModule.vi"("Transmit Frame in"=w704, "Numeric"=1, "Numeric 2"=6) -> ("Transmit Frame out"=w703:T3)  [unwired: 8 in]
              }
            }
          }
        }
        n92 = feedback-in #1(w383) -> ()
        n93 = Unbundle By Name(w446) -> ("data[0]"=w255:u8, "data[2]"=w254:u8, "data[3]"=w253:u8, "data[4]"=w410:u8, "data[5]"=w386:u8, "data[6]"=w409:u8, "data[7]"=w408:u8)  [unwired: 1 out]
        n94 = Equal?(x=u32 273, y=w387) -> (x = y?=w252:bool)
        n95 = Equal?(x=u32 1297, y=w387) -> (x = y?=w407:bool)
        n96 = Equal?(x=w387, y=u32 1041) -> (x = y?=w406:bool)
        n97 = Equal?(x=w255, y=u8 1) -> (x = y?=w421:bool)
        "MOD 1" <- w421
        n98 = Equal?(x=w255, y=u8 3) -> (x = y?=w419:bool)
        "MOD 3" <- w419
        n99 = Equal?(x=w255, y=u8 4) -> (x = y?=w411:bool)
        "MOD 4" <- w411
        n100 = Equal?(x=w255, y=u8 5) -> (x = y?=w391:bool)
        "MOD 5" <- w391
        n101 = Equal?(x=w255, y=u8 6) -> (x = y?=w390:bool)
        "MOD 6" <- w390
        n102 = Equal?(x=w255, y=u8 2) -> (x = y?=w420:bool)
        "MOD 2" <- w420
        n103 = shared-variable "SBU-cRIO\\Variables for FPGA V4.lvlib\\Transmit Frame"(w453) -> ()  [unwired: 1 in, 1 out]
        n104 = shared-variable "SBU-cRIO\\Variables for FPGA V4.lvlib\\Transmit"(w447) -> ()  [unwired: 1 in, 1 out]
        n105 = feedback #2() -> (w440:dbl)
        n106 = feedback #3() -> (w439:dbl)
        n107 = feedback #4() -> (w441:dbl)
        n108 = feedback #5() -> (w438:dbl)
        n109 = feedback #6() -> (w437:dbl)
        n110 = feedback #7() -> (w436:dbl)
        n111 = feedback #8() -> (w429:dbl)
        n112 = feedback #9() -> (w430:dbl)
        n113 = feedback #10() -> (w431:dbl)
        n114 = call "CAP-MOD-1.vi"("Boolean 3"=w421, "data[2]"=w254, "Numeric 7"=w436, "data[3]"=w253, "data[4]"=w410, "data[5]"=w386, "data[6]"=w409, "Boolean"=w406, "data[7]"=w408, "Boolean 2"=w407, "Count per volt"=w247, "Numeric 10"=w439, "Numeric 9"=w438, "Numeric 11"=w440, "Numeric 8"=w437, "Numeric 12"=w441) -> ("Numeric 5"=w349:dbl, "Numeric 4"=w348:dbl, "Numeric 6"=w351:dbl, "Numeric"=w345:dbl, "Numeric 3"=w347:dbl, "Numeric 2"=w346:dbl)  [unwired: 6 in]
        "TAP 1_1" <- w351
        "TAP 1_2" <- w349
        "TAP 1_3" <- w348
        "TAP 1_4" <- w347
        "TAP 1_5" <- w346
        "TAP 1_6" <- w345
        n115 = feedback-in #2(w349) -> ()
        n116 = feedback-in #3(w348) -> ()
        n117 = feedback-in #4(w351) -> ()
        n118 = feedback-in #5(w347) -> ()
        n119 = feedback-in #6(w346) -> ()
        n120 = feedback-in #7(w345) -> ()
        n121 = feedback #11() -> (w434:dbl)
        n122 = feedback #12() -> (w433:dbl)
        n123 = feedback #13() -> (w432:dbl)
        n124 = call "CAP-MOD-4.vi"("Count per volt"=w247, "Boolean 3"=w420, "Numeric 10"=w432, "data[2]"=w254, "data[3]"=w253, "data[4]"=w410, "data[5]"=w386, "Boolean"=w406, "data[6]"=w409, "Boolean 2"=w407, "data[7]"=w408, "Numeric 9"=w431, "Numeric 12"=w434, "Numeric 8"=w430, "Numeric 11"=w433, "Numeric 7"=w429) -> ("Numeric 4"=w325:dbl, "Numeric 5"=w326:dbl, "Numeric 6"=w327:dbl, "Numeric 3"=w324:dbl, "Numeric"=w322:dbl, "Numeric 2"=w323:dbl)  [unwired: 6 in]
        "TAP 2_1" <- w327
        "TAP 2_2" <- w326
        "TAP 2_3" <- w325
        "TAP 2_4" <- w324
        "TAP 2_5" <- w323
        "TAP 2_6" <- w322
        n125 = feedback-in #8(w327) -> ()
        n126 = feedback-in #9(w326) -> ()
        n127 = feedback-in #10(w325) -> ()
        n128 = feedback-in #11(w324) -> ()
        n129 = feedback-in #12(w323) -> ()
        n130 = feedback-in #13(w322) -> ()
        n131 = feedback #14() -> (w425:dbl)
        n132 = feedback #15() -> (w427:dbl)
        n133 = feedback #16() -> (w426:dbl)
        n134 = feedback #17() -> (w424:dbl)
        n135 = feedback #18() -> (w422:dbl)
        n136 = feedback #19() -> (w423:dbl)
        n137 = call "CAP-M0D3.vi"("data[2]"=w254, "data[3]"=w253, "Numeric 8"=w423, "data[4]"=w410, "data[5]"=w386, "data[6]"=w409, "data[7]"=w408, "Boolean"=w406, "Count per volt"=w247, "Boolean 2"=w407, "Boolean 3"=w419, "Numeric 10"=w425, "Numeric 9"=w424, "Numeric 11"=w426, "Numeric 7"=w422, "Numeric 12"=w427) -> ("Numeric 5"=w302:dbl, "Numeric 4"=w301:dbl, "Numeric 6"=w303:dbl, "Numeric 3"=w300:dbl, "Numeric 2"=w299:dbl, "Numeric"=w298:dbl)  [unwired: 6 in]
        "TAP 3_4" <- w300
        "TAP 3_5" <- w299
        "TAP 3_6" <- w298
        "TAP 3_1" <- w303
        "TAP 3_2" <- w302
        "TAP 3_3" <- w301
        n138 = feedback-in #14(w301) -> ()
        n139 = feedback-in #15(w303) -> ()
        n140 = feedback-in #16(w302) -> ()
        n141 = feedback-in #17(w300) -> ()
        n142 = feedback-in #18(w299) -> ()
        n143 = feedback-in #19(w298) -> ()
        n144 = feedback #20() -> (w416:dbl)
        n145 = feedback #21() -> (w417:dbl)
        n146 = feedback #22() -> (w418:dbl)
        n147 = feedback #23() -> (w413:dbl)
        n148 = feedback #24() -> (w412:dbl)
        n149 = feedback #25() -> (w414:dbl)
        n150 = call "CAP-5.vi"("data[2]"=w254, "data[3]"=w253, "Numeric 9"=w414, "Count per volt"=w247, "data[4]"=w410, "data[5]"=w386, "data[6]"=w409, "Boolean"=w406, "data[7]"=w408, "Boolean 2"=w407, "Boolean 3"=w411, "Numeric 12"=w418, "Numeric 8"=w413, "Numeric 11"=w417, "Numeric 7"=w412, "Numeric 10"=w416) -> ("Numeric 5"=w278:dbl, "Numeric 4"=w277:dbl, "Numeric 6"=w370:dbl, "Numeric 3"=w276:dbl, "Numeric 2"=w275:dbl, "Numeric"=w274:dbl)  [unwired: 6 in]
        "TAP 4_1" <- w278
        "TAP 4_2" <- w277
        "TAP 4_3" <- w370
        "TAP 4_" <- w276
        "TAP 20" <- w275
        "TAP 19" <- w274
        n151 = feedback-in #20(w278) -> ()
        n152 = feedback-in #21(w277) -> ()
        n153 = feedback-in #22(w370) -> ()
        n154 = feedback-in #23(w276) -> ()
        n155 = feedback-in #24(w275) -> ()
        n156 = feedback-in #25(w274) -> ()
        n157 = feedback #26() -> (w394:dbl)
        n158 = feedback #27() -> (w393:dbl)
        n159 = feedback #28() -> (w392:dbl)
        n160 = feedback #29() -> (w397:dbl)
        n161 = feedback #30() -> (w396:dbl)
        n162 = feedback #31() -> (w395:dbl)
        n163 = call "CAP-MOD-5.vi"("data[2]"=w254, "data[3]"=w253, "Numeric 10"=w395, "data[4]"=w410, "data[5]"=w386, "data[6]"=w409, "data[7]"=w408, "Boolean 2"=w406, "Count per volt"=w247, "Boolean 3"=w407, "Boolean"=w391, "Numeric 9"=w394, "Numeric 12"=w397, "Numeric 8"=w393, "Numeric 11"=w396, "Numeric 7"=w392) -> ("Numeric 6"=w369:dbl, "Numeric 5"=w368:dbl, "Numeric 4"=w367:dbl, "Numeric 3"=w366:dbl, "Numeric 2"=w365:dbl, "Numeric"=w364:dbl)  [unwired: 6 in]
        "TAP 18" <- w369
        "TAP 17" <- w368
        "TAP 16" <- w367
        "TAP 15" <- w366
        "TAP 14" <- w365
        "TAP 13" <- w364
        n164 = feedback-in #26(w369) -> ()
        n165 = feedback-in #27(w368) -> ()
        n166 = feedback-in #28(w367) -> ()
        n167 = feedback-in #29(w366) -> ()
        n168 = feedback-in #30(w365) -> ()
        n169 = feedback-in #31(w364) -> ()
        n170 = feedback #32() -> (w400:dbl)
        n171 = feedback #33() -> (w399:dbl)
        n172 = feedback #34() -> (w398:dbl)
        n173 = feedback #35() -> (w403:dbl)
        n174 = feedback #36() -> (w402:dbl)
        n175 = feedback #37() -> (w401:dbl)
        n176 = call "CAP-MOD-6.vi"("data[2]"=w254, "data[3]"=w253, "Numeric 10"=w401, "data[4]"=w410, "data[5]"=w386, "Count per volt"=w247, "data[6]"=w409, "Boolean 2"=w406, "data[7]"=w408, "Boolean 3"=w407, "Boolean"=w390, "Numeric 7"=w398, "Numeric 12"=w403, "Numeric 8"=w399, "Numeric 11"=w402, "Numeric 9"=w400) -> ("Numeric 6"=w363:dbl, "Numeric 5"=w362:dbl, "Numeric 4"=w361:dbl, "Numeric 3"=w360:dbl, "Numeric 2"=w359:dbl, "Numeric"=w358:dbl)  [unwired: 6 in]
        "TAP 12" <- w363
        "TAP 11" <- w362
        "TAP 10" <- w361
        "TAP 9" <- w360
        "TAP 8" <- w359
        "TAP 7" <- w358
        n177 = feedback-in #32(w363) -> ()
        n178 = feedback-in #33(w362) -> ()
        n179 = feedback-in #34(w361) -> ()
        n180 = feedback-in #35(w360) -> ()
        n181 = feedback-in #36(w359) -> ()
        n182 = feedback-in #37(w358) -> ()
        n183 = case shown="1, Default" w255 {
          tunnel: w252 -> [w574 w585 w596 w607 w618 w629]
          tunnel: w386 -> [w573 w584 w595 w606 w617 w628]
          tunnel: [w572 w586 w598 w608 w622 w634] -> w385
          tunnel: w384 -> [w571 w586 w598 w608 w622 w634]
          tunnel: [w570 w583 w597 w609 w621 w633] -> w380
          tunnel: w379 -> [w570 w582 w597 w609 w621 w633]
          tunnel: [w569 w581 w594 w610 w620 w632] -> w377
          tunnel: w378 -> [w569 w581 w593 w610 w620 w632]
          tunnel: [w568 w580 w592 w605 w619 w631] -> w375
          tunnel: w376 -> [w568 w580 w592 w604 w619 w631]
          tunnel: [w567 w579 w591 w603 w616 w630] -> w374
          tunnel: w373 -> [w567 w579 w591 w603 w615 w630]
          tunnel: [w566 w578 w590 w602 w614 w627] -> w372
          tunnel: w371 -> [w566 w578 w590 w602 w614 w626]
          frame 1, Default {
            n184 = case shown="True" w574 {
              tunnel: w573 -> [_ w577]
              tunnel: [w575 w576] -> w572
              tunnel: w571 -> [w575 _]
              frame False {
              }
              frame True {
                n185 = To Double Precision Float(number=w577) -> (double precision float=w576:dbl)
              }
            }
          }
          frame 2 {
            n186 = case shown="True" w585 {
              tunnel: w584 -> [_ w589]
              tunnel: [w587 w588] -> w583
              tunnel: w582 -> [w587 _]
              frame False {
              }
              frame True {
                n187 = To Double Precision Float(number=w589) -> (double precision float=w588:dbl)
              }
            }
          }
          frame 3 {
            n188 = case shown="True" w596 {
              tunnel: w595 -> [_ w601]
              tunnel: [w599 w600] -> w594
              tunnel: w593 -> [w599 _]
              frame False {
              }
              frame True {
                n189 = To Double Precision Float(number=w601) -> (double precision float=w600:dbl)
              }
            }
          }
          frame 4 {
            n190 = case shown="True" w607 {
              tunnel: w606 -> [_ w613]
              tunnel: [w611 w612] -> w605
              tunnel: w604 -> [w611 _]
              frame False {
              }
              frame True {
                n191 = To Double Precision Float(number=w613) -> (double precision float=w612:dbl)
              }
            }
          }
          frame 5 {
            n192 = case shown="True" w618 {
              tunnel: w617 -> [_ w625]
              tunnel: [w623 w624] -> w616
              tunnel: w615 -> [w623 _]
              frame False {
              }
              frame True {
                n193 = To Double Precision Float(number=w625) -> (double precision float=w624:dbl)
              }
            }
          }
          frame 6 {
            n194 = case shown="False" w629 {
              tunnel: w628 -> [_ w637]
              tunnel: [w635 w636] -> w627
              tunnel: w626 -> [w635 _]
              frame False {
              }
              frame True {
                n195 = To Double Precision Float(number=w637) -> (double precision float=w636:dbl)
              }
            }
          }
        }
        "Temp_1" <- w385
        "Temp_2" <- w380
        "Temp_3" <- w377
        "Temp_4" <- w375
        "Temp_5" <- w374
        "Temp_6" <- w372
        n196 = Build Array(w351, w349, w348, w347, w346, w345, w327, w326, w325, w324, w323, w322, w303, w302, w301, w300, w299, w298, w278, w277, w370, w276, w275, w274, w369, w368, w367, w366, w365, w364, w363, w362, w361, w360, w359, w358) -> (w357:dbl[])
        n197 = call "Elapsed Time"("Time Target (s)"=w354, "Auto Reset"=TRUE) -> ()  [unwired: 10 in, 8 out]
        n198 = Add(x=w354, y=w352) -> (x+y=w353:dbl)
        n199 = Array To Cluster(array=w357) -> ()  [unwired: 1 out]
        n200 = case shown="5" w255 {
          tunnel: w254 -> [w465 w487 w509 w531 w553]
          tunnel: w253 -> [w464 w486 w508 w530 w552]
          tunnel: w252 -> [w463 w485 w507 w529 w551]
          tunnel: w251 -> [w462 w484 w506 w528 w550]
          tunnel: [w461 w484 w506 w528 w550] -> w243
          tunnel: [w460 w483 w505 w527 w549] -> w242
          tunnel: w250 -> [w460 w482 w505 w527 w549]
          tunnel: [w459 w481 w504 w526 w548] -> w241
          tunnel: w249 -> [w459 w481 w503 w526 w548]
          tunnel: [w458 w480 w502 w525 w544] -> w240
          tunnel: w248 -> [w458 w480 w502 w524 w544]
          tunnel: w247 -> [w457 w479 w501 w523 w547]
          tunnel: [w456 w478 w500 w522 w546] -> w239
          tunnel: w246 -> [w456 w478 w500 w522 w545]
          frame 1, Default {
            n201 = case shown="True" w463 {
              tunnel: [w466 w470] -> w461
              tunnel: w465 -> [_ w469]
              tunnel: w464 -> [_ w468]
              tunnel: w462 -> [w466 _]
              tunnel: w457 -> [_ w467]
              frame False {
              }
              frame True {
                n202 = To Double Precision Float(number=w469) -> (double precision float=w472:dbl)
                n203 = To Double Precision Float(number=w468) -> (double precision float=w471:dbl)
                n204 = Multiply(x=w471, y=255.0) -> (x*y=w474:dbl)
                n205 = Add(x=w472, y=w474) -> (x+y=w476:dbl)
                n206 = Multiply(x=w476, y=w467) -> (x*y=w475:dbl)
                n207 = Divide(x=w475, y=1000.0) -> (x/y=w470:dbl)
              }
            }
          }
          frame 2 {
            n208 = case shown="True" w485 {
              tunnel: [w488 w492] -> w483
              tunnel: w487 -> [_ w491]
              tunnel: w486 -> [_ w490]
              tunnel: w482 -> [w488 _]
              tunnel: w479 -> [_ w489]
              frame False {
              }
              frame True {
                n209 = To Double Precision Float(number=w491) -> (double precision float=w494:dbl)
                n210 = To Double Precision Float(number=w490) -> (double precision float=w493:dbl)
                n211 = Multiply(x=w493, y=255.0) -> (x*y=w496:dbl)
                n212 = Add(x=w494, y=w496) -> (x+y=w498:dbl)
                n213 = Multiply(x=w498, y=w489) -> (x*y=w497:dbl)
                n214 = Divide(x=w497, y=1000.0) -> (x/y=w492:dbl)
              }
            }
          }
          frame 3 {
            n215 = case shown="True" w507 {
              tunnel: w509 -> [_ w514]
              tunnel: w508 -> [_ w513]
              tunnel: [w510 w512] -> w504
              tunnel: w503 -> [w510 _]
              tunnel: w501 -> [_ w511]
              frame False {
              }
              frame True {
                n216 = To Double Precision Float(number=w514) -> (double precision float=w516:dbl)
                n217 = To Double Precision Float(number=w513) -> (double precision float=w515:dbl)
                n218 = Multiply(x=w515, y=255.0) -> (x*y=w518:dbl)
                n219 = Add(x=w516, y=w518) -> (x+y=w520:dbl)
                n220 = Multiply(x=w520, y=w511) -> (x*y=w519:dbl)
                n221 = Divide(x=w519, y=1000.0) -> (x/y=w512:dbl)
              }
            }
          }
          frame 4 {
            n222 = case shown="True" w529 {
              tunnel: w531 -> [_ w536]
              tunnel: w530 -> [_ w535]
              tunnel: [w532 w534] -> w525
              tunnel: w524 -> [w532 _]
              tunnel: w523 -> [_ w533]
              frame False {
              }
              frame True {
                n223 = To Double Precision Float(number=w536) -> (double precision float=w538:dbl)
                n224 = To Double Precision Float(number=w535) -> (double precision float=w537:dbl)
                n225 = Multiply(x=w537, y=255.0) -> (x*y=w540:dbl)
                n226 = Add(x=w538, y=w540) -> (x+y=w542:dbl)
                n227 = Multiply(x=w542, y=w533) -> (x*y=w541:dbl)
                n228 = Divide(x=w541, y=1000.0) -> (x/y=w534:dbl)
              }
            }
          }
          frame 5 {
            n229 = case shown="True" w551 {
              tunnel: w553 -> [_ w558]
              tunnel: w552 -> [_ w557]
              tunnel: w547 -> [_ w556]
              tunnel: [w554 w555] -> w546
              tunnel: w545 -> [w554 _]
              frame False {
              }
              frame True {
                n230 = To Double Precision Float(number=w558) -> (double precision float=w560:dbl)
                n231 = To Double Precision Float(number=w557) -> (double precision float=w559:dbl)
                n232 = Multiply(x=w559, y=255.0) -> (x*y=w562:dbl)
                n233 = Add(x=w560, y=w562) -> (x+y=w564:dbl)
                n234 = Multiply(x=w564, y=w556) -> (x*y=w563:dbl)
                n235 = Divide(x=w563, y=1000.0) -> (x/y=w555:dbl)
              }
            }
          }
        }
        "VOLT-CAP-1" <- w243
        "VOLT-CAP-2" <- w242
        "VOLT-CAP-3" <- w241
        "VOLT-CAP-4" <- w240
        "VOLT-CAP-5" <- w239
        "Vertical Progress Bar 2" <- w242
        "Vertical Progress Bar 5" <- w239
        "Vertical Progress Bar 4" <- w240
        "Vertical Progress Bar 3" <- w241
        "Vertical Progress Bar" <- w243
        n236 = Build Array (concatenate)(w297, w298) -> (w291:dbl[])
        n237 = Build Array (concatenate)(w296, w299) -> (w290:dbl[])
        n238 = Build Array (concatenate)(w295, w300) -> (w289:dbl[])
        n239 = Build Array (concatenate)(w294, w301) -> (w288:dbl[])
        n240 = Build Array (concatenate)(w356, w352) -> (w279:dbl[])
        n241 = Build Array (concatenate)(w293, w302) -> (w287:dbl[])
        n242 = Build Array (concatenate)(w292, w303) -> (w286:dbl[])
        n243 = Build Array (concatenate)(w350, w351) -> (w333:dbl[])
        n244 = Build Array (concatenate)(w344, w349) -> (w332:dbl[])
        n245 = Build Array (concatenate)(w343, w348) -> (w331:dbl[])
        n246 = Build Array (concatenate)(w342, w347) -> (w330:dbl[])
        n247 = Build Array (concatenate)(w315, w327) -> (w309:dbl[])
        n248 = Build Array (concatenate)(w314, w326) -> (w308:dbl[])
        n249 = Build Array (concatenate)(w341, w346) -> (w329:dbl[])
        n250 = Build Array (concatenate)(w340, w345) -> (w328:dbl[])
        n251 = Build Array (concatenate)(w313, w325) -> (w307:dbl[])
        n252 = Build Array (concatenate)(w312, w324) -> (w306:dbl[])
        n253 = Build Array (concatenate)(w311, w323) -> (w305:dbl[])
        n254 = Build Array (concatenate)(w310, w322) -> (w304:dbl[])
        n255 = Build Array (concatenate)(w273, w278) -> (w261:dbl[])
        n256 = Build Array (concatenate)(w272, w277) -> (w260:dbl[])
        n257 = Build Array (concatenate)(w271, w276) -> (w259:dbl[])
        n258 = Build Array (concatenate)(w270, w275) -> (w258:dbl[])
        n259 = Build Array (concatenate)(w269, w274) -> (w257:dbl[])
        n260 = Build Array (concatenate)(w268, w274) -> (w256:dbl[])
        n261 = Bundle(w279, w291) -> (w285:cluster{dbl[], dbl[]})  [unwired: 1 in]
        n262 = Bundle(w279, w290) -> (w284:cluster{dbl[], dbl[]})  [unwired: 1 in]
        n263 = Bundle(w279, w289) -> (w283:cluster{dbl[], dbl[]})  [unwired: 1 in]
        n264 = Bundle(w279, w288) -> (w282:cluster{dbl[], dbl[]})  [unwired: 1 in]
        n265 = Bundle(w279, w287) -> (w281:cluster{dbl[], dbl[]})  [unwired: 1 in]
        n266 = Bundle(w279, w286) -> (w280:cluster{dbl[], dbl[]})  [unwired: 1 in]
        n267 = Bundle(w279, w333) -> (w339:cluster{dbl[], dbl[]})  [unwired: 1 in]
        n268 = Bundle(w279, w332) -> (w338:cluster{dbl[], dbl[]})  [unwired: 1 in]
        n269 = Bundle(w279, w331) -> (w337:cluster{dbl[], dbl[]})  [unwired: 1 in]
        n270 = Bundle(w279, w330) -> (w336:cluster{dbl[], dbl[]})  [unwired: 1 in]
        n271 = Bundle(w279, w309) -> (w321:cluster{dbl[], dbl[]})  [unwired: 1 in]
        n272 = Bundle(w279, w308) -> (w320:cluster{dbl[], dbl[]})  [unwired: 1 in]
        n273 = Bundle(w279, w329) -> (w335:cluster{dbl[], dbl[]})  [unwired: 1 in]
        n274 = Bundle(w279, w328) -> (w334:cluster{dbl[], dbl[]})  [unwired: 1 in]
        n275 = Bundle(w279, w307) -> (w319:cluster{dbl[], dbl[]})  [unwired: 1 in]
        n276 = Bundle(w279, w306) -> (w318:cluster{dbl[], dbl[]})  [unwired: 1 in]
        n277 = Bundle(w279, w305) -> (w317:cluster{dbl[], dbl[]})  [unwired: 1 in]
        n278 = Bundle(w279, w304) -> (w316:cluster{dbl[], dbl[]})  [unwired: 1 in]
        n279 = Bundle(w279, w261) -> (w267:cluster{dbl[], dbl[]})  [unwired: 1 in]
        n280 = Bundle(w279, w260) -> (w266:cluster{dbl[], dbl[]})  [unwired: 1 in]
        n281 = Bundle(w279, w259) -> (w265:cluster{dbl[], dbl[]})  [unwired: 1 in]
        n282 = Bundle(w279, w258) -> (w264:cluster{dbl[], dbl[]})  [unwired: 1 in]
        n283 = Bundle(w279, w257) -> (w263:cluster{dbl[], dbl[]})  [unwired: 1 in]
        n284 = Bundle(w279, w256) -> (w262:cluster{dbl[], dbl[]})  [unwired: 1 in]
        n285 = Build Array(w339, w338, w337, w336, w335, w334, w321, w320, w319, w318, w317, w316, w285, w284, w283, w282, w281, w280, w267, w266, w265, w264, w263, w262) -> (→"TAP Voltages":cluster{dbl[], dbl[]}[])
        n286 = node-c288() -> ()  [unwired: 1 in, 1 out]
      }
      n287 = VISA Close(VISA resource name=w37, error in (no error)=w36) -> ()  [unwired: 1 out]
      n288 = call <vilib>:"CloseHandle.vi"("client handle"=w23, "error in (no error)"=w22) -> ()  [unwired: 13 in, 1 out]
      n289 = call <vilib>:"CloseHandle.vi"("client handle"=w21, "error in (no error)"=w20) -> ()  [unwired: 13 in, 1 out]
      n290 = node-c288(w66) -> ()  [unwired: 1 out]
    }
  }
